vi "LIA Simulation FPGA on Host.vi"() -> ()   [LabVIEW 2017]
uses:
  <instrlib>/_niInstr/Data Trigger/v1/Shared/Public/Edge Configuration FXP(+-,18,1).ctl
  <instrlib>/_niInstr/Data Trigger/v1/Shared/Public/Edge Configuration Trigger Slope.ctl
  <instrlib>/_niInstr/DSP/v1/Shared/Public/IQ Data.ctl
  <vilib>/Analysis/4window.llb/windowTd.ctl
  <instrlib>/_niInstr/DSP/v1/FPGA/Public/Sub VIs/Frequency Shift/Frequency Shift - 1 spc.vi
  <vilib>/measure/maspectr.llb/FFT Power Spectrum and PSD for 1 Chan.vi
  <instrlib>/_niInstr/DSP/v1/Xnodes/Public/Frequency Shift/niInstr DSP v1 Frequency Shift FPGA.xnode
  <instrlib>/_niInstr/DSP/v1/Shared/niInstr DSP v1 Shared.lvlib
  <instrlib>/_niInstr/DSP/v1/FPGA/niInstr DSP v1 FPGA.lvlib
  <vilib>/addons/Digital Filter Design/NI_DigFilterLicensed.lvlib
  <vilib>/addons/Digital Filter Design/Multirate.llb/DFD MRate Filtering (Array).vi
  <vilib>/ptbypt/NI_PtbyPt.lvlib
  <vilib>/measure/NI_MAPro.lvlib
  <vilib>/Analysis/NI_AALPro.lvlib
  <instrlib>/_niInstr/Data Trigger/v1/Shared/niInstr Data Trigger v1 Shared.lvlib
panel:
  in  "signal freq":dbl=100000.0 format="%#_6p"
  out "# samples":dbl format="%#_f"
  in  "decimating factor":i32=1000
  in  "Tab Control":enum32{"PLL", "Lock-In Signal", "CIC"}(tab)
  out "Accumulator":dbl format="%_12f"
  out "Frequency (f/Fs)":dbl format="%_12f"
  out "Frequency (f/Fs) Graph":dbl(graph)
  out "r":dbl(graph)
  out "I":dbl(graph)
  out "Q":dbl(graph)
  out "Waveform Graph 2":cluster{"f0":dbl, "df":dbl, "magnitude":dbl[]}(graph)
  out "max - min":dbl format="%#_p"
  out "min":dbl
  out "max":dbl
  out "Waveform Graph 1":cluster{"f0":dbl, "df":dbl, "values":dbl[]}[](graph)
  out "I CIC":dbl[][](graph)
  in  "Delay Time (s)":dbl=0.0001 format="%#_13g"
  out "Lock-In Source":dbl(graph)
  out "PLL Source":dbl(graph)
  in  "cic.reset":bool
  out "progress":dbl(slide) scale=0.0..1.0
  in  "lock-in.reset":bool
  in  "lock-in.enable":bool
  in  "stop":bool
  in  "pll.arm":bool
  in  "pll.m":i8=-20
  in  "pll.config":T1={"highLevel"=0.25, "lowLevel"=0.0, "trigger slope"=enum."Positive"}
  in  "pll.reset":bool
  in  "file path":path=path "C:/Repositories/Lock-In-Amplifier/tmds/raw-adc-data-00.tdms"
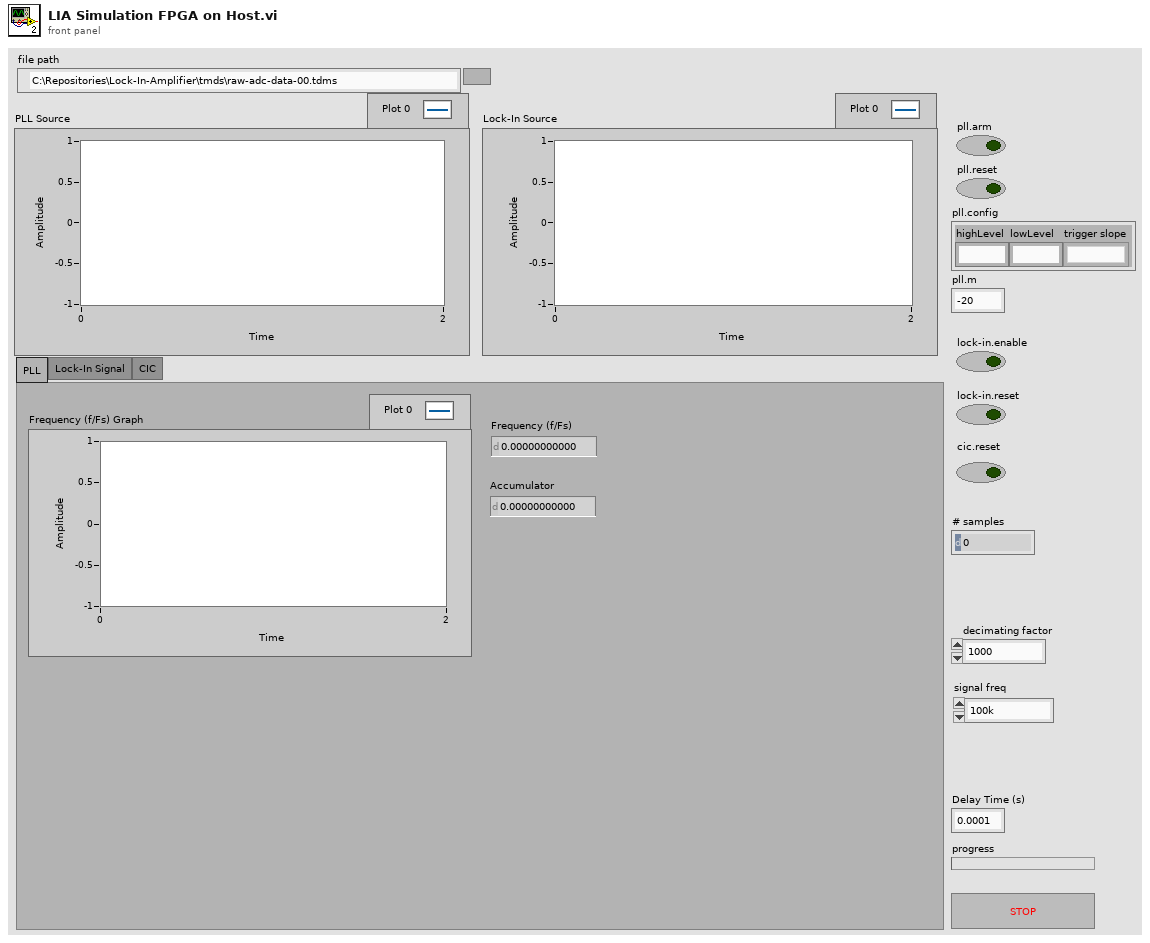
[diagram p1: front panel]
types:
  T1 = typedef "niInstr Data Trigger v1 Shared.lvlib/Edge Configuration FXP(+-,18,1).ctl" = cluster{"highLevel":fxp<+/-,18,1>, "lowLevel":fxp<+/-,18,1>, "trigger slope":T2}
  T2 = typedef "niInstr Data Trigger v1 Shared.lvlib/Edge Configuration Trigger Slope.ctl" = enum8{"Positive", "Negative"}
  T3 = typedef "NI_DigFilterLicensed.lvlib/DFD Multirate Filter Obj.ctl" = cluster{"mMRate_Structure":enum16{"CIC", "FIR", "IIR", "Lattice"}, "mMRate_Mode":T4, "mMRate_Factor":i32, "mMRate_FIRParams":cluster{"mMRate_FIR_H":dbl[], "mMRate_FIR_IsNyquist?":bool, "mMRate_FIR_IsSymmetric?":bool}, "mMRate_CICParams":cluster{"mMRate_CIC_#Stage":i32, "mMRate_CIC_Lag":i32, "mMRate_CIC_Type":enum16{"Lowpass", "Highpass"}}, "mMRate_Order":i32, "mMRate_Version":string, "mMRate_Comments":string, "mMRate_RationalFactor":cluster{"mMRate_L":i32, "mMRate_M":i32}, "mMRate_Fs":dbl, "mMRate_Quantized?":bool, "mMRate_QFilterGain":dbl, "mMRate_CoefWl":i16, "mMRate_Scaling":cluster{"mMRate_ScaleByPowerOf2?":bool, "mMRate_ScaleType":T5}, "mMRate_InputWl":i16, "mMRate_OutputWl":i16, "mMRate_OutputMode":T6, "mMRate_MultMode":T7, "mMRate_BitPruning":bool, "mMRate_GainWl":i16, "mMRate_OutputFwl":i16, "mMRate_SumIwl":i16, "mMRate_InputIwl ":i16, "mMRate_SumWl":i16, "mMRate_CoefIwl":i16}
  T4 = typedef "NI_DigFilterLicensed.lvlib/DFD Multirate Mode.ctl" = i16
  T5 = typedef "NI_DigFilterLicensed.lvlib/DFD Coef Norm Type.ctl" = enum16{"No Norm", "Time Domain 1-Norm", "Time Domain 2-Norm", "Time Domain Inf-Norm"}
  T6 = typedef "NI_DigFilterLicensed.lvlib/DFD Round-off Mode.ctl" = enum16{"Nearest", "Truncation"}
  T7 = typedef "NI_DigFilterLicensed.lvlib/DFD FXP MRate Multiply Mode.ctl" = enum16{"Truncated", "Full"}
  T8 = typedef "niInstr DSP v1 Shared.lvlib/IQ Data.ctl" = cluster{"I":fxp<+/-,18,1>, "Q":fxp<+/-,18,1>, "overflow":bool}
  T9 = typedef "NI_AALPro.lvlib/windowTd.ctl" = u32
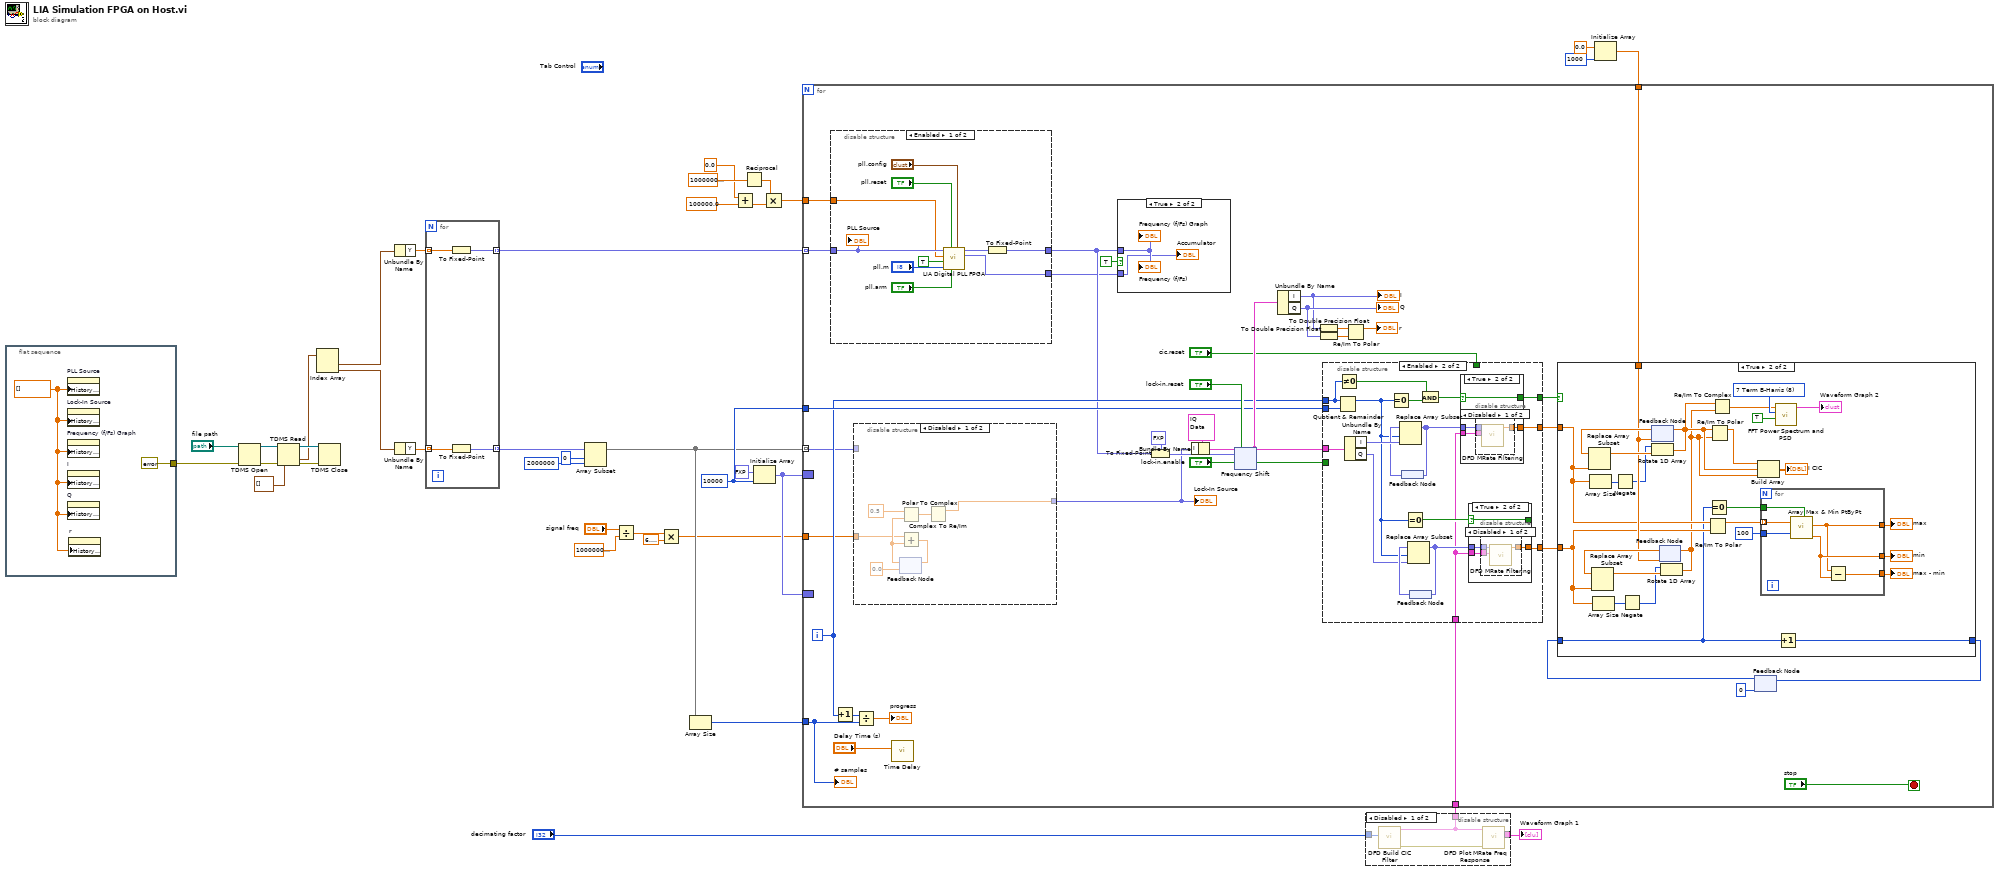
[diagram p0: block diagram]
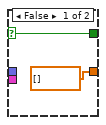
[diagram p8: hidden frame]
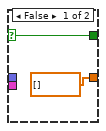
[diagram p10: hidden frame]
diagram:
  w16 = 10000 ("dimension size")
  n1 = flat-sequence {
    tunnel: [errorcluster {"status"=FALSE, "code"=0, "source"=""} ("error constant")] -> w24
    frame #0 {
      w39 = dbl[] [] ("History Data")
      n2 = property on="PLL Source" class="WFChart (strict)"("History Data"=w39) -> ()  [unwired: 2 in, 2 out]
      n3 = property on="Lock-In Source" class="WFChart (strict)"("History Data"=w39) -> ()  [unwired: 2 in, 2 out]
      n4 = property on="Frequency (f/Fs) Graph" class="WFChart (strict)"("History Data"=w39) -> ()  [unwired: 2 in, 2 out]
      n5 = property on="I" class="WFChart (strict)"("History Data"=w39) -> ()  [unwired: 2 in, 2 out]
      n6 = property on="Q" class="WFChart (strict)"("History Data"=w39) -> ()  [unwired: 2 in, 2 out]
      n7 = property on="r" class="WFChart (strict)"("History Data"=w39) -> ()  [unwired: 2 in, 2 out]
    }
  }
  n8 = TDMS Open(8:w24, 11:"file path") -> (0:w36:errorcluster, 3:w37:refnum<k34>)  [unwired: 5 in]
  n9 = TDMS Read(0:w37, 11:w36, 12:waveform(dbl)[] []) -> (4:w34:refnum<k34>, 10:w32:waveform(dbl)[], 15:w33:errorcluster)  [unwired: 5 in, 3 out]
  n10 = Index Array(array=w32) -> (element #1=w31:waveform(dbl), element #2=w28:waveform(dbl))  [unwired: 2 in]
  n11 = TDMS Close(8:w33, 11:w34) -> ()  [unwired: 2 out]
  n12 = Unbundle By Name(w31) -> ("Y"=w30:dbl[])
  n13 = Unbundle By Name(w28) -> ("Y"=w29:dbl[])
  n14 = for {
    tunnel: w30 -> [w44] mode=indexing
    tunnel: [w43] -> w27 mode=indexing
    tunnel: w29 -> [w42] mode=indexing
    tunnel: [w41] -> w26 mode=indexing
    n15 = To Fixed-Point(number=w44) -> (fixed-point=w43:fxp<+/-,18,1>)  [unwired: 1 in]
    n16 = To Fixed-Point(number=w42) -> (fixed-point=w41:fxp<+/-,18,1>)  [unwired: 1 in]
  }
  n17 = Array Subset(array=w26, index=0, length=2000000) -> (w11:fxp<+/-,18,1>[])
  n18 = Divide(x="signal freq", y=100000000.0 ("x")) -> (x/y=w6:dbl)
  n19 = Multiply(x=w6, y=6.283185307179586) -> (x*y=w3:dbl)
  n20 = Array Size(array=w11) -> (size(s)=w25:i32)
  n21 = Add(x=0.0, y=100000.0) -> (x+y=w2:dbl)
  n22 = Reciprocal(x=100000000.0) -> (1/x=w22:dbl)
  n23 = Initialize Array(fxp<+/-,18,1> 0.0 ("I"), w16) -> (w12:fxp<+/-,18,1>[])
  n24 = Multiply(x=w22, y=w2) -> (x*y=w20:dbl)
  n25 = disable-structure shown="Disabled" {
    disable-tunnel: [w48 _] -> w19
    disable-tunnel: [w47 _] -> w18
    disable-tunnel: "decimating factor" -> [w45 _]
    frame Disabled {
      n26 = call <vilib>:"DFD Build CIC Filter.vi"("factor"=w45) -> ("error out"=w46:errorcluster, "CIC filter out"=w48:T3)  [unwired: 9 in]
      n27 = call <vilib>:"DFD Plot MRate Freq Response.vi"("error in (no error)"=w46, "multirate filter in"=w48) -> ("magnitude response"=w47:cluster{"f0":dbl, "df":dbl, "values":dbl[]}[])  [unwired: 6 in, 3 out]
    }
    frame Enabled {
    }
  }
  "Waveform Graph 1" <- w18
  n28 = Initialize Array(0.0 ("element"), 1000 ("dimension size")) -> (w14:dbl[])
  n29 = for {
    tunnel: w27 -> [w75] mode=indexing
    tunnel: w11 -> [w51] mode=indexing
    tunnel: w25 -> [w68]
    tunnel: w20 -> [w73]
    tunnel: w19 -> [w67]
    border: w12 -> [_]
    tunnel: w16 -> [w66]
    tunnel: w14 -> [w64]
    border: w12 -> [_]
    tunnel: w3 -> [w53]
    i -> [w65]
    stop <- "stop" stop-if-true
    n30 = disable-structure shown="Enabled" {
      disable-tunnel: w75 -> [w100 _]
      disable-tunnel: [w98 w106] -> w60
      disable-tunnel: w73 -> [w99 w106]
      disable-tunnel: [w96 _] -> w49
      frame Enabled {
        n31 = call "LIA Digital PLL FPGA.vi"("configuration"="pll.config", "arm"="pll.arm", "reset"="pll.reset", "m"="pll.m", "input valid"=TRUE, "q"=w99, "I"=w100) -> ("accumulator"=w96:fxp<+/-,48,0>, "frequency shift"=w97:fxp<+/-,48,0>)  [unwired: 1 in, 2 out]
        n32 = To Fixed-Point(number=w97) -> (fixed-point=w98:fxp<+/-,48,0>)  [unwired: 1 in]
        "PLL Source" <- w100
      }
      frame Disabled {
      }
    }
    n33 = Increment(x=w65) -> (x+1=w80:i32)
    n34 = disable-structure shown="Disabled" {
      disable-tunnel: w53 -> [w88 _]
      disable-tunnel: [w86 w93] -> w50
      disable-tunnel: w51 -> [_ w93]
      frame Disabled {
        n35 = feedback #1(0.0 ("r")) -> (w89:dbl)
        n36 = Polar To Complex(1:w89, 2:0.5 ("r")) -> (0:w87:cdb)
        n37 = Add(x=w88, y=w89) -> (x+y=w90:dbl)
        n38 = feedback-in #1(w90) -> ()
        n39 = Complex To Re/Im(x + iy=w87) -> (x=w86:dbl)  [unwired: 1 out]
      }
      frame Enabled {
      }
    }
    "Lock-In Source" <- w50
    n40 = Divide(x=w80, y=w68) -> (x/y=→"progress":dbl)
    n41 = call "Time Delay"("Delay Time (s)"="Delay Time (s)") -> ()  [unwired: 10 in, 1 out]
    n42 = case shown="True" TRUE {
      tunnel: w60 -> [_ w95]
      tunnel: w49 -> [_ w94]
      frame False {
      }
      frame True {
        "Frequency (f/Fs) Graph" <- w95
        "Frequency (f/Fs)" <- w95
        "Accumulator" <- w94
      }
    }
    n43 = To Fixed-Point(fixed-point type=fxp<+/-,48,0> 0.0 ("frequency shift"), number=w60) -> (fixed-point=w58:fxp<+/-,48,0>)
    n44 = Bundle By Name(cluster=T8 {"I"=0.0, "Q"=0.0, "overflow"=FALSE} ("data"), "I"=w50) -> (w83:T8)
    n45 = xnode "Frequency Shift"("data in"=w83, "reset"="lock-in.reset", "frequency shift"=w58, "input valid"="lock-in.enable") -> ("data out"=w78:T8, "output valid"=w77:bool)  [unwired: 2 in, 1 out]
    n46 = Unbundle By Name(w78) -> ("I"=w52:fxp<+/-,18,1>, "Q"=w70:fxp<+/-,18,1>)
    "I" <- w52
    "Q" <- w70
    n47 = To Double Precision Float(number=w52) -> (double precision float=w72:dbl)
    n48 = To Double Precision Float(number=w70) -> (double precision float=w71:dbl)
    n49 = disable-structure shown="Enabled" {
      disable-tunnel: w78 -> [_ w158]
      disable-tunnel: w77 -> [_ _]
      disable-tunnel: "cic.reset" -> [_ _]
      disable-tunnel: w67 -> [_ w145]
      disable-tunnel: w65 -> [_ w142]
      disable-tunnel: w66 -> [_ w157]
      disable-tunnel: [_ w151] -> w63
      disable-tunnel: [_ w152] -> w62
      disable-tunnel: [_ w144] -> w57
      frame Disabled {
      }
      frame Enabled {
        n50 = Quotient & Remainder(x=w142, y=w157) -> (x-y*floor(x/y)=w147:i32)  [unwired: 1 out]
        n51 = Not Equal To 0?(x=w142) -> (x != 0?=w141:bool)
        n52 = Unbundle By Name(w158) -> ("I"=w156:fxp<+/-,18,1>, "Q"=w146:fxp<+/-,18,1>)
        n53 = Equal To 0?(x=w147) -> (x = 0?=w154:bool)
        n54 = feedback #2() -> (w155:fxp<+/-,18,1>[])
        n55 = Replace Array Subset(array=w155, new element=w156, index=w147) -> (w153:fxp<+/-,18,1>[])
        n56 = feedback-in #2(w153) -> ()
        n57 = Equal To 0?(x=w147) -> (x = 0?=w149:bool)
        n58 = feedback #3() -> (w148:fxp<+/-,18,1>[])
        n59 = Replace Array Subset(array=w148, new element=w146, index=w147) -> (w150:fxp<+/-,18,1>[])
        n60 = feedback-in #3(w150) -> ()
        n61 = And(x=w141, y=w154) -> (x .and. y?=w143:bool)
        n62 = case shown="True" w143 {
          selector: w143 -> [w169 w170]
          tunnel: w145 -> [_ w173]
          tunnel: w153 -> [_ w172]
          tunnel: [dbl[] [] ("signal out") w171] -> w151
          tunnel: [w169 w170] -> w152
          frame False {
          }
          frame True {
            n63 = disable-structure shown="Disabled" {
              disable-tunnel: w173 -> [w176 _]
              disable-tunnel: w172 -> [w175 _]
              disable-tunnel: [w174 _] -> w171
              frame Disabled {
                n64 = call-poly <vilib>:"DFD MRate Filtering.vi"("multirate filter"=w176, "signal in"=w175) -> ("signal out"=w174:dbl[])  [unwired: 8 in, 1 out]
              }
              frame Enabled {
              }
            }
          }
        }
        n65 = case shown="True" w149 {
          selector: w149 -> [w160 w161]
          tunnel: w145 -> [_ w164]
          tunnel: w150 -> [_ w163]
          tunnel: [dbl[] [] ("signal out") w162] -> w144
          tunnel: [w160 w161] -> _
          frame False {
          }
          frame True {
            n66 = disable-structure shown="Disabled" {
              disable-tunnel: w164 -> [w167 _]
              disable-tunnel: w163 -> [w166 _]
              disable-tunnel: [w165 _] -> w162
              frame Disabled {
                n67 = call-poly <vilib>:"DFD MRate Filtering.vi"("multirate filter"=w167, "signal in"=w166) -> ("signal out"=w165:dbl[])  [unwired: 8 in, 1 out]
              }
              frame Enabled {
              }
            }
          }
        }
      }
    }
    n68 = Re/Im To Polar(2:w71, 3:w72) -> (1:→"r":dbl)  [unwired: 1 out]
    n69 = feedback #4(u64 0 ("index")) -> (w55:u64)
    n70 = case shown="True" w62 {
      tunnel: w64 -> [_ w128]
      tunnel: w63 -> [_ w123]
      tunnel: w57 -> [_ w122]
      tunnel: w55 -> [w107 w116]
      tunnel: [w107 w117] -> w56
      frame False {
      }
      frame True {
        w113 = T9 8 items=["Rectangle"=0, "Hanning"=1, "Hamming"=2, "Blackman-Harris"=3, "Exact Blackman"=4, "Blackman"=5, "Flat Top"=6, "4 Term B-Harris "=7, "7 Term B-Harris"=8, "Low Sidelobe"=9, "Blackman Nuttall"=11, "Triangle"=30, "Bartlett-Hanning"=31, "Bohman"=32, "Parzen"=33, "Welch"=34, "Kaiser"=60, "Dolph-Chebyshev"=61, "Gaussian"=62] ("window")
        n71 = Array Size(array=w123) -> (size(s)=w133:i32)
        n72 = Array Size(array=w122) -> (size(s)=w130:i32)
        n73 = Negate(x=w133) -> (-x=w126:i32)
        n74 = Negate(x=w130) -> (-x=w125:i32)
        n75 = feedback #5(w128) -> (w132:dbl[])
        n76 = Replace Array Subset(array=w132, new element=w123) -> (w134:dbl[])  [unwired: 1 in]
        n77 = Rotate 1D Array(1:w134, 2:w126) -> (0:w111:dbl[])
        n78 = feedback-in #5(w111) -> ()
        n79 = feedback #6(w128) -> (w131:dbl[])
        n80 = Replace Array Subset(array=w131, new element=w122) -> (w129:dbl[])  [unwired: 1 in]
        n81 = Rotate 1D Array(1:w129, 2:w125) -> (0:w110:dbl[])
        n82 = feedback-in #6(w110) -> ()
        n83 = Re/Im To Polar(2:w122, 3:w123) -> (1:w118:dbl[])  [unwired: 1 out]
        n84 = Equal To 0?(x=w116) -> (x = 0?=w115:bool)
        n85 = Re/Im To Polar(2:w110, 3:w111) -> (1:w112:dbl[])  [unwired: 1 out]
        n86 = Re/Im To Complex(1:w110, 2:w111) -> (0:w109:cdb[])
        n87 = Build Array(w112, w111, w110) -> (→"I CIC":dbl[][])
        n88 = for {
          tunnel: [w140] -> w124
          tunnel: 100 ("sample length") -> [w139]
          tunnel: [w138] -> w120
          tunnel: [w137] -> w119
          tunnel: w118 -> [w136] mode=indexing
          tunnel: w115 -> [w135]
          n89 = call <vilib>:"Array Max & Min PtByPt.vi"("input data point"=w136, "sample length"=w139, "initialize"=w135) -> ("max value"=w137:dbl, "min value"=w138:dbl)  [unwired: 3 out]
          n90 = Subtract(x=w137, y=w138) -> (x-y=w140:dbl)
        }
        "min" <- w120
        "max - min" <- w124
        "max" <- w119
        n91 = call-poly <vilib>:"FFT Power Spectrum and PSD.vi"("dB On (F)"=TRUE, "window"=w113, "time signal"=w109) -> ("Power Spectrum / PSD"=→"Waveform Graph 2":cluster{"f0":dbl, "df":dbl, "magnitude":dbl[]})  [unwired: 5 in, 3 out]
        n92 = Increment(x=w116) -> (x+1=w117:u64)
      }
    }
    n93 = feedback-in #4(w56) -> ()
    "# samples" <- w68
  }
